vi "FPGACompileStatus.vi"(11 "targetVIref":refnum<vi>) -> (0 "error out":errorcluster, 1 "timed out":bool, 3 "compile done":bool)   [LabVIEW 2020, in "NI_TargetHelper.lvlib"]
uses:
  <vilib>/TargetSupport/NI_TargetHelper/NI_TargetHelper.lvlib
  <vilib>/rvi/CDR/niFpgaBuild_JobState.ctl
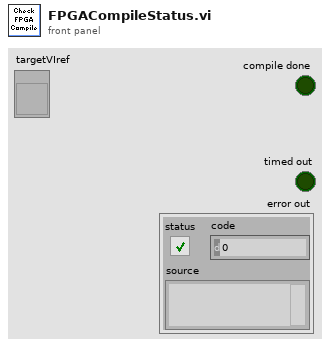
[diagram p1: front panel]
types:
  T1 = typedef "niFpgaBuild_JobState.ctl" = enum16{"Waiting", "Working", "Cancelled", "Complete", "Error"}
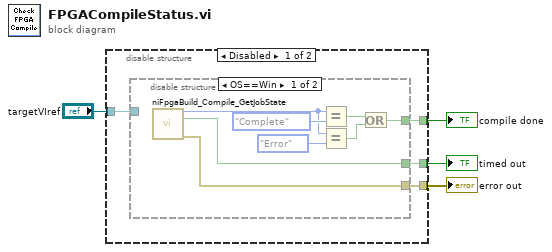
[diagram p0: block diagram]
diagram:
  n1 = disable-structure shown="Disabled" {
    disable-tunnel: "targetVIref" -> [w8 _]
    disable-tunnel: [w7 _] -> w3
    disable-tunnel: [w6 _] -> w2
    disable-tunnel: [w5 _] -> w1
    frame Disabled {
      n2 = disable-structure shown="OS==Win" {
        disable-tunnel: w8 -> [_ _]
        disable-tunnel: [w16 _] -> w7
        disable-tunnel: [w15 _] -> w6
        disable-tunnel: [w9 _] -> w5
        frame condition #0 {
          n3 = call <vilib>:"niFpgaBuild_Compile_GetJobState.vi"() -> ("job state"=w10:T1, "timed out"=w16:bool, "error out"=w15:errorcluster)  [unwired: 13 in]
          n4 = Equal?(x=w10, y=niFpgaBuild_JobState."Complete") -> (x = y?=w12:bool)
          n5 = Equal?(x=w10, y=niFpgaBuild_JobState."Error") -> (x = y?=w11:bool)
          n6 = Or(x=w12, y=w11) -> (x .or. y?=w9:bool)
        }
        frame condition #1 (active) {
        }
      }
    }
    frame Enabled {
    }
  }
  "timed out" <- w3
  "error out" <- w2
  "compile done" <- w1
